vi "simulated_g=1.2.vi"() -> ()   [LabVIEW 2016]
panel:
  out "trion 2":cluster{dbl[], dbl[]}[](graph)
  out "pair 2":cluster{dbl[], dbl[]}[](graph)
  out "widths":cluster{dbl[], dbl[]}[](graph)
  out "amplitudes":cluster{dbl[], dbl[]}[](graph)
  in  "trion":cluster{dbl[], dbl[]}(graph)={[3.25, 3.5, 3.75, 4.0, 4.25, 4.5, 4.75, 5.0, 5.25, 5.5, 5.75, 6.0, 6.25, 6.5, 6.75, 7.0], [0.11363104635575436, 0.09838018138197059, 0.08703448533097628, 0.07439457342612806, 0.06141965475908567, 0.04977211561594542, 0.044832191560037454, 0.029985318879672093, 0.03943751158223989, 0.03604536607443924, 0.04844719894329341, 0.05975932191490109, 0.07219804240169153, 0.08527330487321857, 0.09873590391091787, 0.1124410277274705]}
  in  "pair":cluster{dbl[], dbl[]}(graph)={[2.5, 2.75, 3.0, 3.25, 3.5, 3.75, 4.0, 4.25, 4.5, 4.75, 5.0, 5.25, 5.5, 5.75, 6.0, 6.25, 6.5, 6.75], [0.08733288160751611, 0.07920374335619833, 0.06632326743073644, 0.05477506926461709, 0.042641717611656575, 0.030520942159979452, 0.01762461850315068, 0.010346602956210722, 0.007738869226157318, 0.02565246638735947, 0.025455964764332022, 0.04537705286527765, 0.0542443424130359, 0.067510310719439, 0.07973801035870007, 0.09196432090154123, 0.10419065113262688, 0.11641691529446005]}
  in  "fits 2":cluster{dbl[], dbl[]}[](graph)
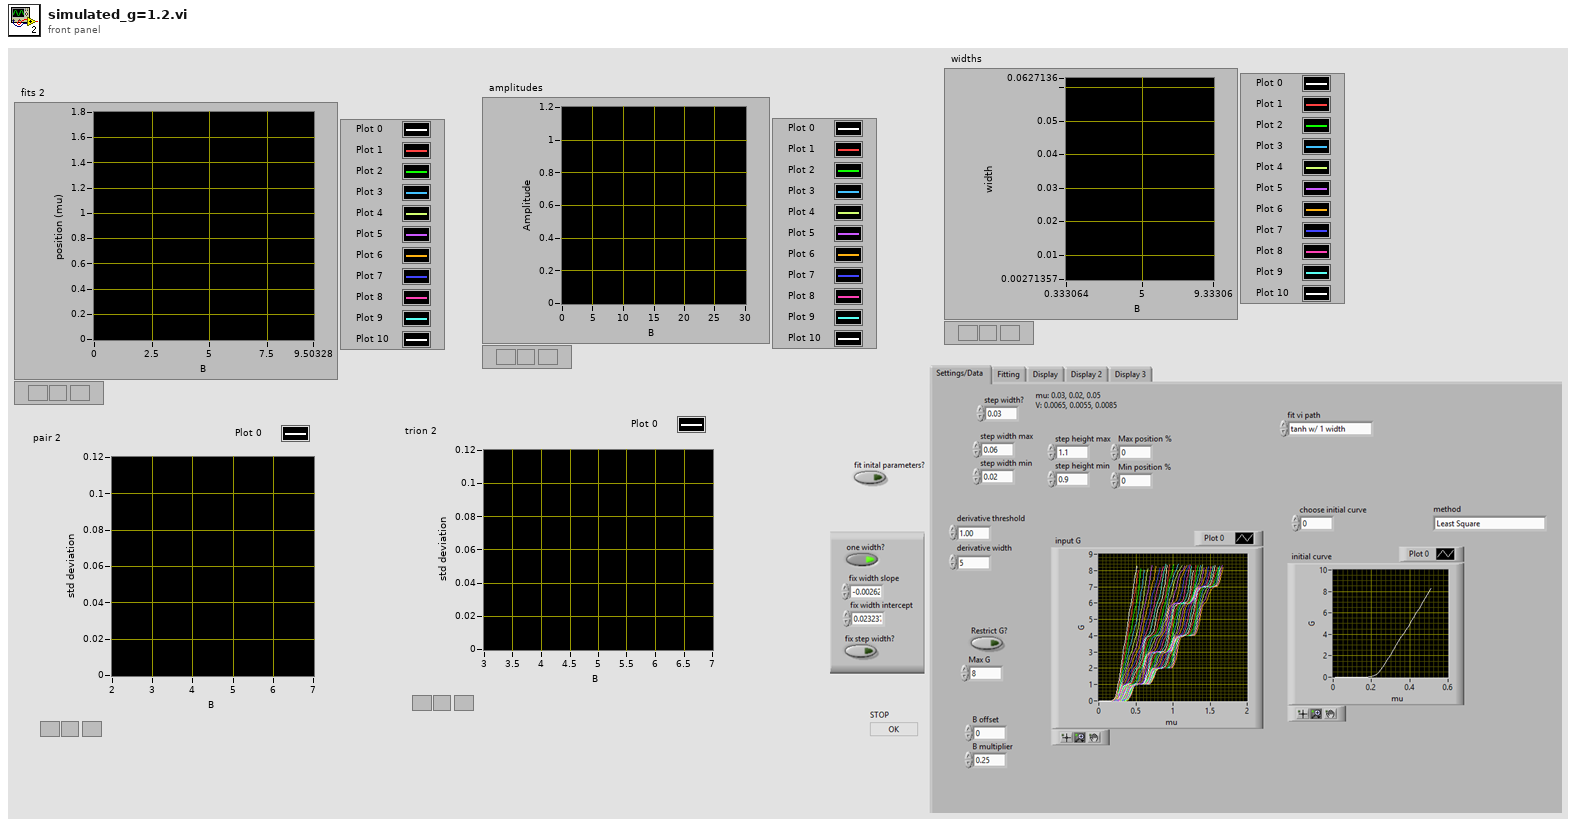
[diagram p1: front panel]
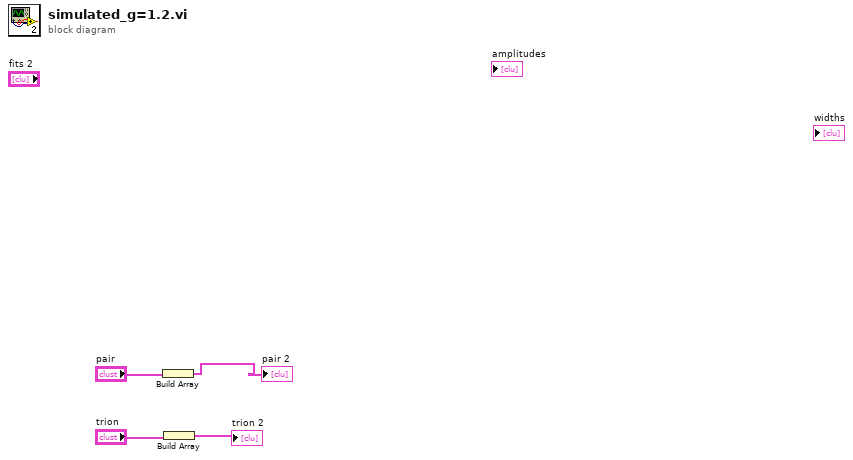
[diagram p0: block diagram]
diagram:
  n1 = Build Array("pair") -> (→"pair 2":cluster{dbl[], dbl[]}[])
  n2 = Build Array("trion") -> (→"trion 2":cluster{dbl[], dbl[]}[])
